vi "sub_simluation_count.vi"(7 "cmd":enum16{"ini", "count"}(ring)=enum."count", 11 "data":u32) -> (2 "current":u32, 3 "max":dbl)   [LabVIEW 2016]
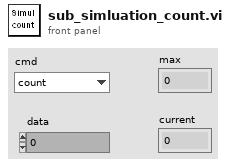
[diagram p1: front panel]
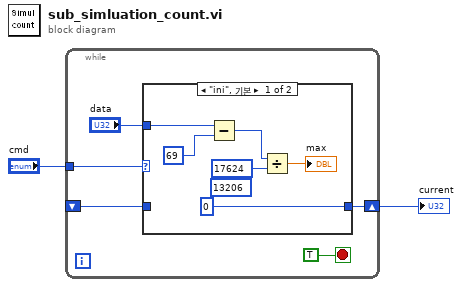
[diagram p0: block diagram]
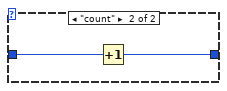
[diagram p2: hidden frame]
diagram:
  n1 = while {
    tunnel: "cmd" -> [w6]
    shift-right: [w5] -> w1
    shift-left: _ -> [w3]
    stop <- TRUE stop-if-true
    n2 = case shown="\"ini\", 기본" w6 {
      tunnel: [u32 0 w14] -> w5
      tunnel: "data" -> [w12 _]
      tunnel: w3 -> [_ w15]
      frame "ini", Default {
        (unwired) u32 13206 ("y")
        n3 = Subtract(x=w12, y=u32 69) -> (x-y=w10:u32)
        n4 = Divide(x=w10, y=u32 17624) -> (x/y=→"max":dbl)
      }
      frame "count" {
        n5 = Increment(x=w15) -> (x+1=w14:u32)
      }
    }
  }
  "current" <- w1
